vi "Main_WSC.vi"() -> ()   [LabVIEW 2019]
uses:
  WSCbot_V3_Toolkit.lvlibp
panel:
  out "Error Out":errorcluster
  in  "Error In":errorcluster
  in  "move to see arror":cluster{"X":dbl, "Y":dbl, "Z":dbl}[](array[cluster])=[{"X"=-7.0, "Y"=15.0, "Z"=-35.0}]
  out "Stop Output":bool=TRUE
  in  "Stop Button":bool
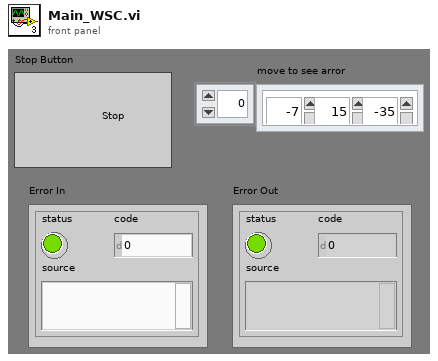
[diagram p1: front panel]
types:
  T1 = enum16{"Right_up", "Right_down", "Left_down", "Left_up", "left", "right", "up", "down"}
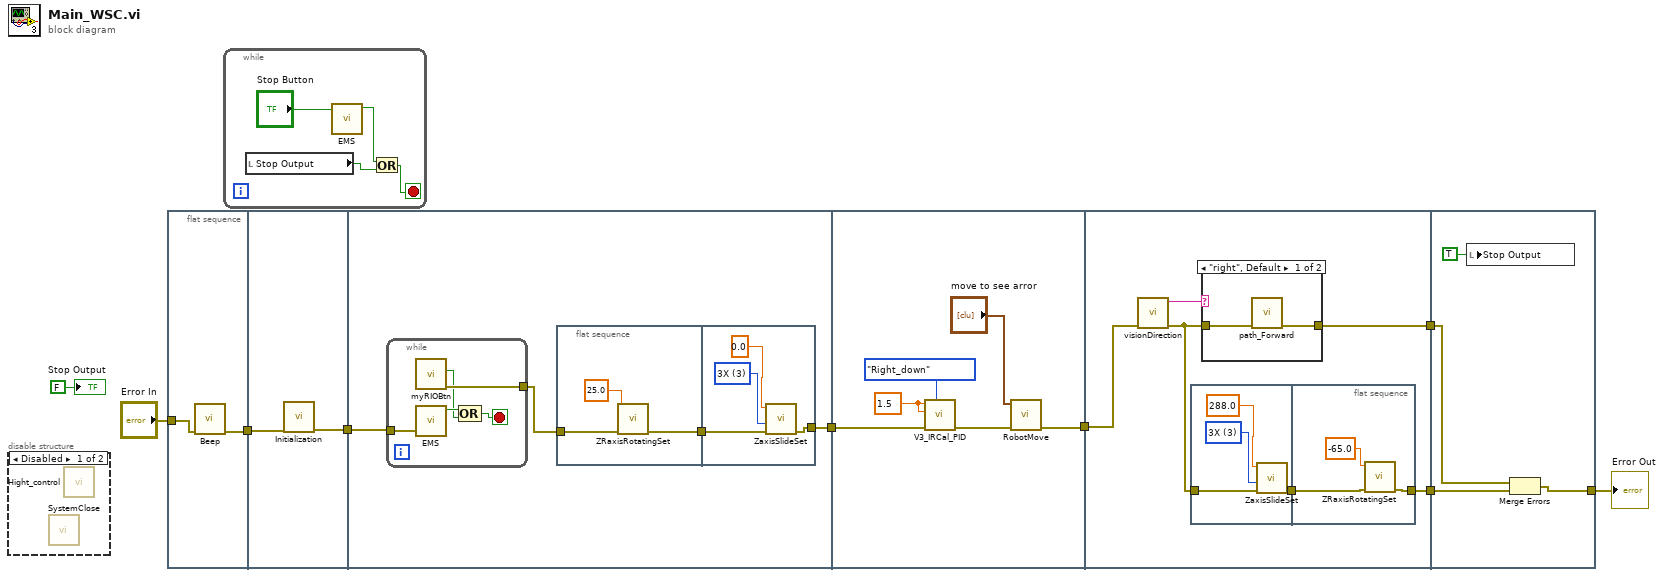
[diagram p0: block diagram]
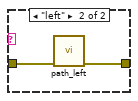
[diagram p3: hidden frame]
diagram:
  n1 = disable-structure shown="Disabled" {
    frame Disabled {
      n2 = call "SystemClose.vi"() -> ()  [unwired: 3 in, 1 out]
      n3 = call "Hight_control.vi"() -> ()  [unwired: 11 in, 1 out]
    }
    frame Enabled {
    }
  }
  n4 = flat-sequence {
    tunnel: [w11] -> w5
    tunnel: "Error In" -> [w10]
    tunnel: [w13] -> w6
    tunnel: w5 -> [w12]
    tunnel: [w16] -> w7
    tunnel: w6 -> [w15]
    tunnel: [w35] -> w8
    tunnel: w7 -> [w30]
    tunnel: w8 -> [w39]
    tunnel: [w37] -> w3
    tunnel: [w36] -> w1
    tunnel: w3 -> [w54]
    tunnel: [w55] -> w2
    tunnel: w1 -> [w53]
    frame #0 {
      n5 = call "Beep.vi"("Error In"=w10) -> ("Error Out"=w11:errorcluster)  [unwired: 10 in]
    }
    frame #1 {
      n6 = call "Initialization.vi"("Error In"=w12) -> ("Error Out"=w13:errorcluster)  [unwired: 10 in]
    }
    frame #2 {
      n7 = while {
        tunnel: [w29] -> w17
        tunnel: w15 -> [w25]
        stop <- w26 stop-if-true
        n8 = call "myRIOBtn.vi"() -> ("error out"=w29:errorcluster, "myRIOButton"=w27:bool)  [unwired: 10 in]
        n9 = call "EMS.vi"("error in"=w25) -> ("EMS"=w28:bool)  [unwired: 9 in, 1 out]
        n10 = Compound Arithmetic op=OR(w28, w27) -> (w26:bool)
      }
      n11 = flat-sequence {
        tunnel: w17 -> [w19]
        tunnel: [w18] -> w14
        tunnel: w14 -> [w22]
        tunnel: [w21] -> w16
        frame #0 {
          n12 = call "ZRaxisRotatingSet.vi"("error in"=w19, "TargetHight(deg)"=25.0) -> ("error out"=w18:errorcluster)  [unwired: 8 in, 1 out]
        }
        frame #1 {
          w24 = u16 3 items=["0X", "1X", "2X", "3X"] ("findHomeVel (times)")
          n13 = call "ZaxisSlideSet.vi"("error in"=w22, "findHomeVel (times)"=w24, "TargetABSHight(mm)"=0.0) -> ("error out"=w21:errorcluster)  [unwired: 7 in, 1 out]
        }
      }
    }
    frame #3 {
      w31 = 1.5 ("X_distance(V)")
      n14 = call "V3_IRCal_PID.vi"("Direction"=T1."Right_down", "Error In"=w30, "Y_distance(V)"=w31, "X_distance(V)"=w31) -> ("Error Out"=w33:errorcluster)  [unwired: 6 in, 1 out]
      n15 = call "RobotMove.vi"("error in (no error)"=w33, "XYZ"="move to see arror") -> ("error out"=w35:errorcluster)  [unwired: 9 in]
    }
    frame #4 {
      n16 = call "visionDirection.vi"("Error In"=w39) -> ("Error Out"=w38:errorcluster, "Direction"=w41:string)  [unwired: 9 in]
      n17 = flat-sequence {
        tunnel: [w45] -> w40
        tunnel: w38 -> [w42]
        tunnel: w40 -> [w48]
        tunnel: [w46] -> w37
        frame #0 {
          w44 = u16 3 items=["0X", "1X", "2X", "3X"] ("findHomeVel (times)")
          n18 = call "ZaxisSlideSet.vi"("error in"=w42, "findHomeVel (times)"=w44, "TargetABSHight(mm)"=288.0) -> ("error out"=w45:errorcluster)  [unwired: 7 in, 1 out]
        }
        frame #1 {
          n19 = call "ZRaxisRotatingSet.vi"("error in"=w48, "TargetHight(deg)"=-65.0) -> ("error out"=w46:errorcluster)  [unwired: 8 in, 1 out]
        }
      }
      n20 = case shown="\"right\", Default" w41 {
        tunnel: w38 -> [w50 w52]
        tunnel: [w49 w51] -> w36
        frame "right", Default {
          n21 = call "path_Forward.vi"("Error In"=w50) -> ("Error Out"=w49:errorcluster)  [unwired: 10 in]
        }
        frame "left" {
          n22 = call "path_left.vi"("Error In"=w52) -> ("Error Out"=w51:errorcluster)  [unwired: 10 in]
        }
      }
    }
    frame #5 {
      n23 = local write "Stop Output"(TRUE ("Stop Output")) -> ()
      n24 = Merge Errors(w53, w54) -> (w55:errorcluster)
    }
  }
  n25 = while {
    stop <- w59 stop-if-true
    n26 = local read "Stop Output"() -> (w57:bool)
    n27 = call "EMS.vi"("ProgramStop"="Stop Button") -> ("EMS"=w58:bool)  [unwired: 9 in, 1 out]
    n28 = Or(x=w58, y=w57) -> (x .or. y?=w59:bool)
  }
  "Stop Output" <- FALSE ("Boolean")
  "Error Out" <- w2
